vi "prueba2.vi"() -> ()   [LabVIEW 2016]
uses:
  C:/Users/Polaritones IICO/Desktop/Camara y mapeo/rot/Thorlabs.MotionControl.Controls.dll
  rot/Thorlabs.MotionControl.Controls.dll
  <vilib>/userdefined/High Color/IMAQdx.ctl
  <vilib>/UPVI/lvhdf5/file.llb/LVH5F Operation.ctl
  C:/Users/Polaritones IICO/Desktop/Camara y mapeo/rot/Thorlabs.MotionControl.IntegratedStepperMotorsCLI.dll
  rot/Thorlabs.MotionControl.IntegratedStepperMotorsCLI.dll
  <vilib>/Utility/miscctls.llb/LVRectTypeDef.ctl
  <vilib>/UPVI/lvhdf5/group.llb/H5G_obj_t.ctl
  <vilib>/UPVI/lvhdf5/dataset.llb/LVH5D Operation.ctl
  <vilib>/Analysis/baseanly.llb/Mean (DBL).vi
  <vilib>/UPVI/lvhdf5/group.llb/OpenCreateGroup (String).vi
  <vilib>/UPVI/lvhdf5/utility.llb/Select HDF5 Dialog.vi
  <vilib>/UPVI/lvhdf5/utility.llb/Select HDF5 Dialog (Object Only).vi
  <vilib>/UPVI/lvhdf5/dataset.llb/Simple H5Dwrite (Variant).vi
  <vilib>/UPVI/lvhdf5/library.llb/HDF5 Ref.ctl
  <vilib>/UPVI/lvhdf5/dataset.llb/Simple H5Dwrite.xnode
  <vilib>/vision/driver/NI_Vision_Acquisition_Software.lvlib
  <instrlib>/Keithley 2200 Series/Keithley 2200 Series.lvlib
  <vilib>/Analysis/NI_AALBase.lvlib
  <vilib>/UPVI/lvhdf5/identifier.llb/Not an HDF5 Refnum Constant.vi
  <vilib>/Utility/error.llb/Error Cluster From Error Code.vi
  <vilib>/UPVI/lvhdf5/dataset.llb/OpenCreateReplace Dataset by Element Type.vi
  <vilib>/UPVI/lvhdf5/dataspace.llb/H5Sselect_hyperslab.vi
  <vilib>/UPVI/lvhdf5/dataset.llb/H5Dwrite (Variant).vi
  <vilib>/UPVI/lvhdf5/dataset.llb/H5Dget_space.vi
  <vilib>/UPVI/lvhdf5/attribute.llb/private/LVH5AwriteWDTAttrs.vi
  <vilib>/UPVI/lvhdf5/dataspace.llb/H5Sclose.vi
  <vilib>/UPVI/lvhdf5/dataset.llb/H5Dclose.vi
  <vilib>/UPVI/lvhdf5/utility.llb/Select HDF5 Dialog (File and Object).vi
panel:
  out "valor potenciometro":dbl format="%^#_9e"
  out "Readout string":string
  out "New":bool
  out "Error log":string
  in  "path":path
  out "Ángulo del polarizador":i32
  in  "CageRotatorControl":refnum<k24>(container)
  in  "SerialNumber":string="55000538"
  in  "Ring":u16(ring)
  out "I-V":cluster{dbl[], dbl[]}(graph)
  out "corriente":dbl
  in  "stop medición":bool
  in  "stop":bool
  in  "Iniciar medición":bool
  out "LockIn":dbl
  out "Valor voltaje":dbl
  in  "Config. fotodiodo":cluster{"tiempo. lect.":dbl, "num. med":dbl}
  in  "Powermeter":T1={"Readout Config"="POW", "tiempo. lect."=0.0, "average rate"=0.0}
  in  "config. Polarizador":T2
  in  "Config. voltaje y corriente":T3 {"Measurement Function (0:Voltage)" items=["Voltage", "Current", "Power"]; "Unit(V)" items=["V", "mV", "kV", "A", "mA"]; "Function(0:Voltage)" items=["Voltage", "Current"]}
  in  "yFin":dbl
  in  "Paso":dbl=0.01
  in  "xFin":dbl
  in  "Movimiento de spot en x":ext(slide) scale=-10.0..10.0
  in  "Movimiento de spot en y":dbl(slide) min=-10.0 max=10.0 scale=-10.0..10.0
  out "xsal":dbl
  out "ysal":dbl
  in  "tipo":enum16{"barrido", "manual"}(ring)
  out "Fototubo":cluster{dbl[], dbl[]}(graph)
  out "Power meter":cluster{dbl[], dbl[]}(graph)
  out "Imágen":T4(plugin-control)
  # "Control espejos"
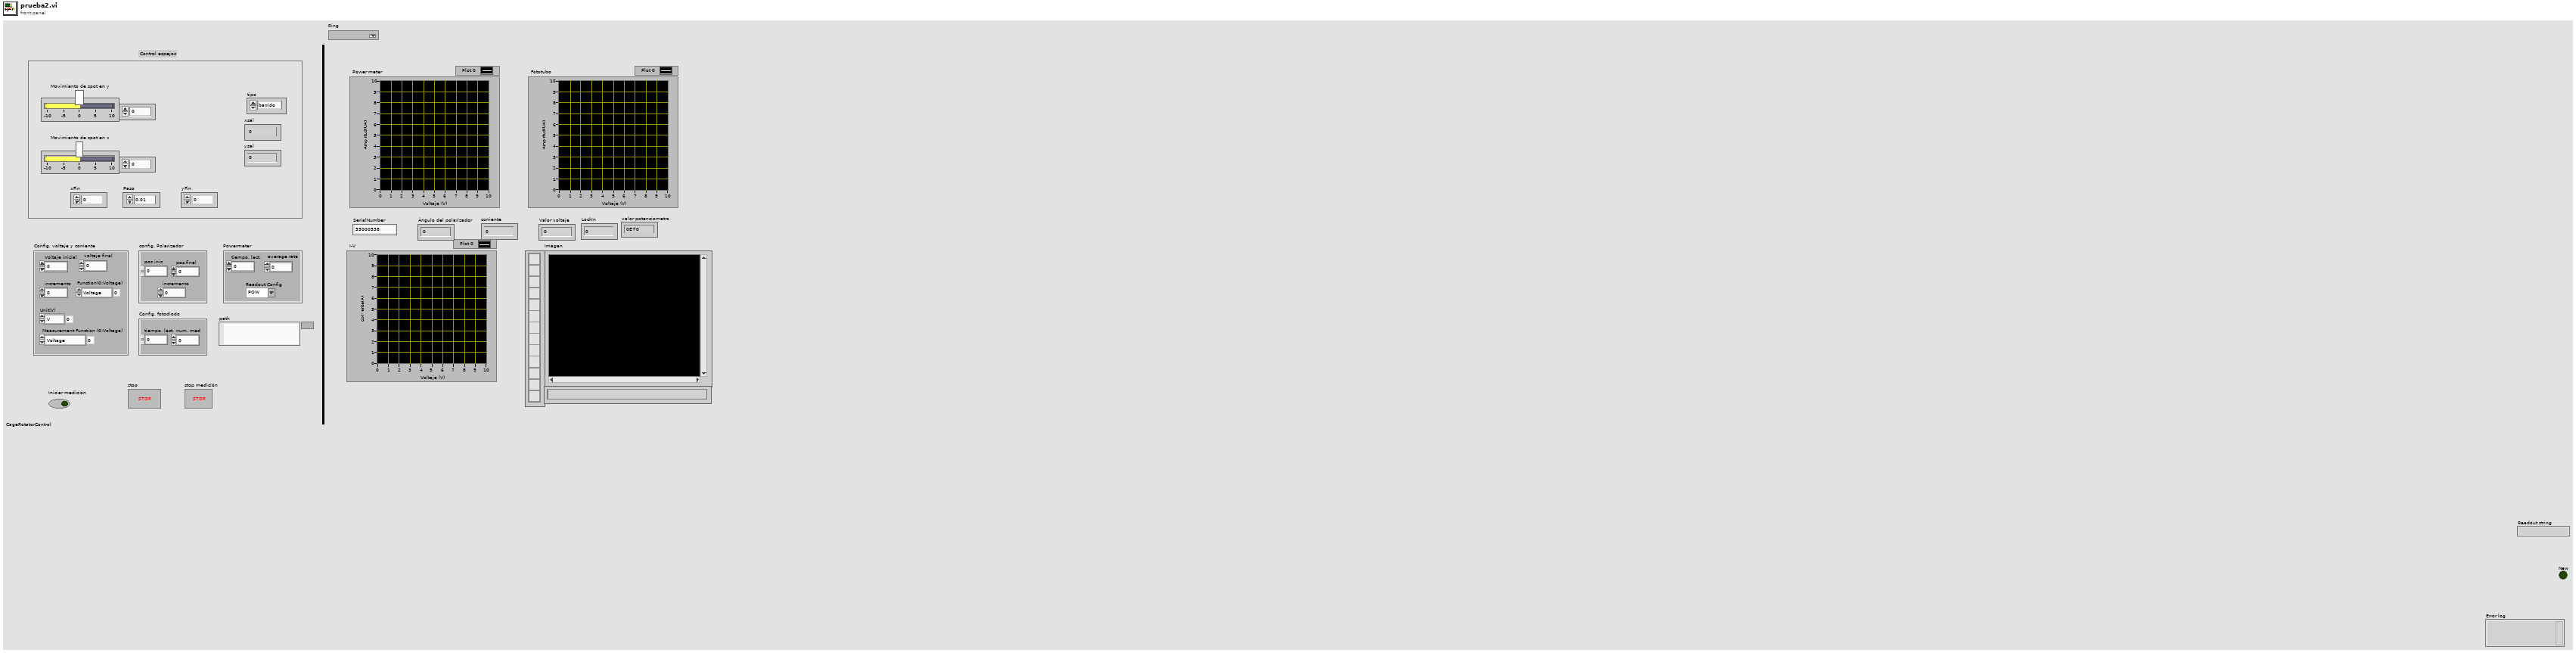
[diagram p1: front panel]
types:
  T1 = cluster{"Readout Config":string, "tiempo. lect.":dbl, "average rate":dbl}
  T2 = cluster{"pos inic":dbl, "pos.final":dbl, "incremento":dbl}
  T3 = cluster{"Voltaje inicial":dbl, "incremento":dbl, " voltaje final":dbl, "Function(0:Voltage)":u16, "Unit(V)":u16, "Measurement Function (0:Voltage)":u16}
  T4 = typedef "IMAQ Image.ctl" = refnum<image>
  T5 = typedef "IMAQdx.ctl" = refnum<k21>
  T6 = typedef "LVH5F Operation.ctl" = enum16{"open", "open or create", "create or replace", "create or replace (with confirmation)", "create", "open (read only)"}
  T7 = typedef "LVRectTypeDef.ctl" = cluster{"Left":i16, "Top":i16, "Right":i16, "Bottom":i16}
  T8 = cluster{"Behavior":enum32{"Invalid", "Default", "Floating", "Floating/Auto-Hide", "Modal"}, "Position":T7, "Center":bool, "Title":string}
  T9 = typedef "LVH5D Operation.ctl" = enum16{"open", "replace", "create", "open or create", "create or replace", "create or replace with confirmation"}
  T10 = typedef "H5G_obj_t.ctl" = i32
  T11 = cluster{"Object Types (any)":T10[], "Object Pattern":string}
  T12 = typedef "Image Type" = u32
  T13 = typedef "HDF5 Ref.ctl" = refnum<k1>
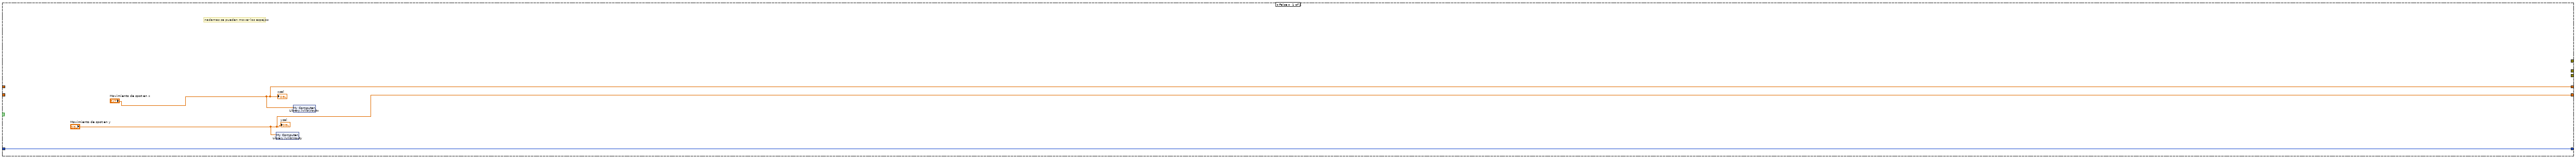
[diagram p2: hidden frame]
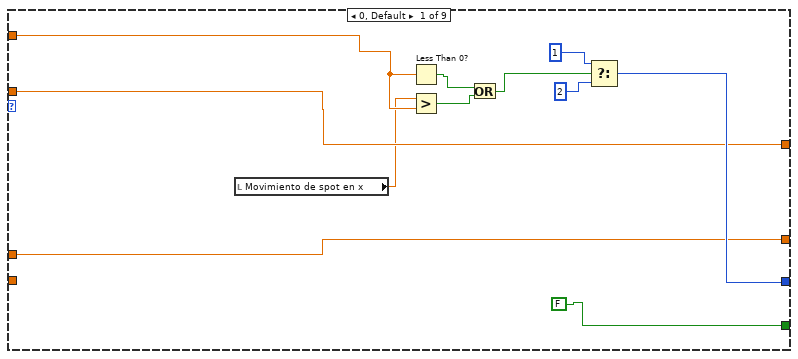
[diagram p3: hidden frame]
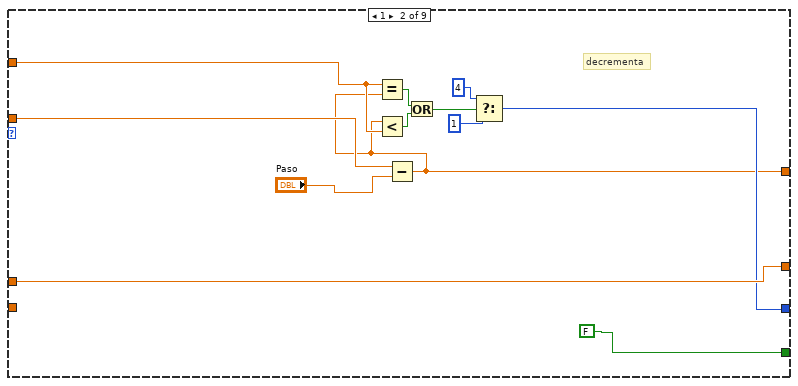
[diagram p4: hidden frame]
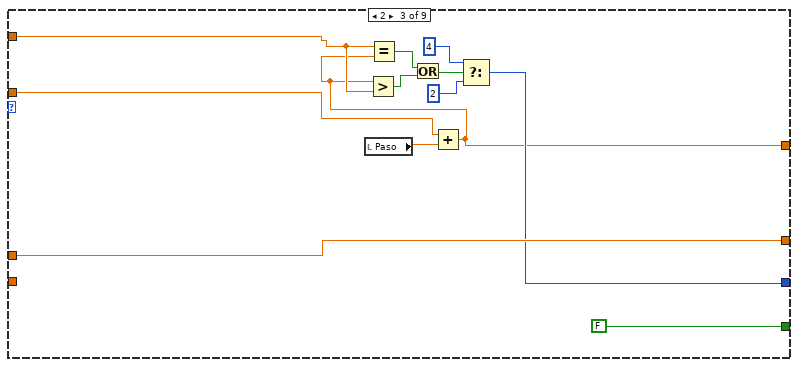
[diagram p5: hidden frame]
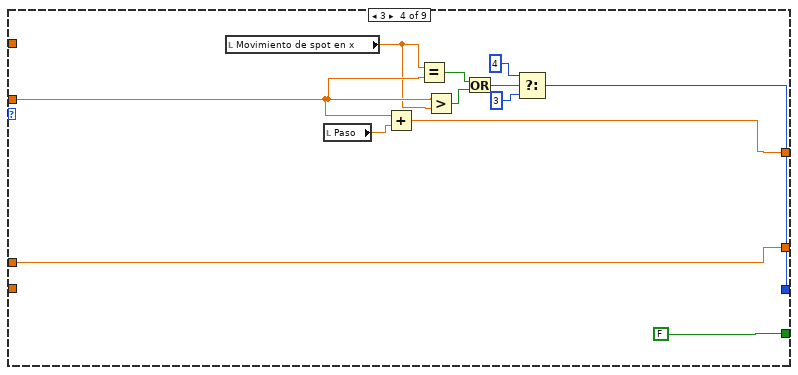
[diagram p6: hidden frame]
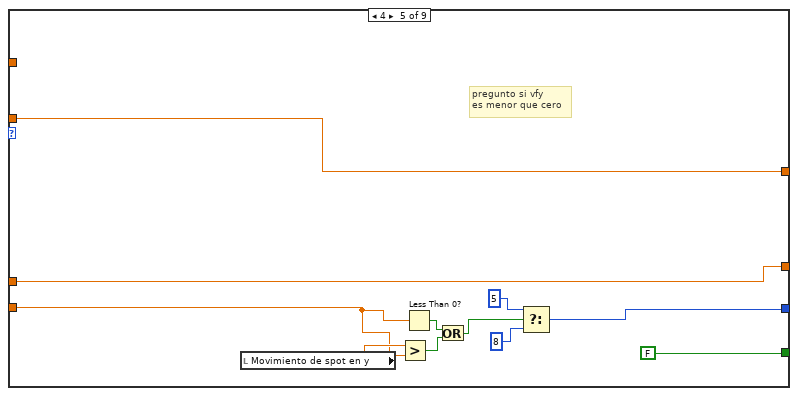
[diagram p7: hidden frame]
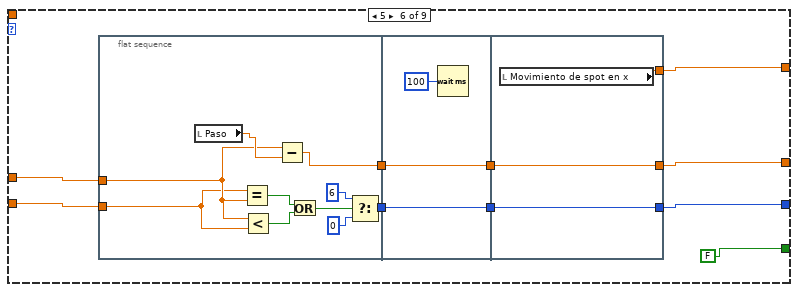
[diagram p8: hidden frame]
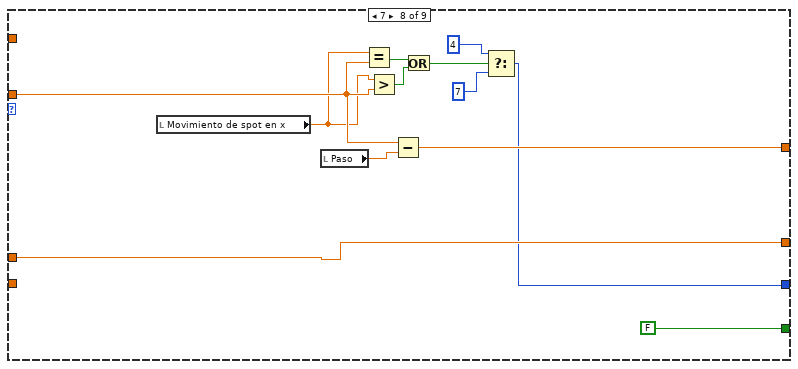
[diagram p9: hidden frame]
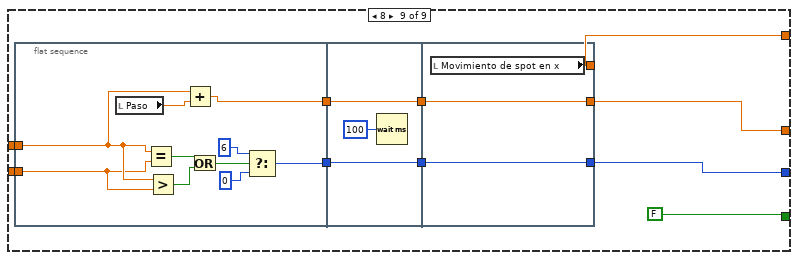
[diagram p10: hidden frame]
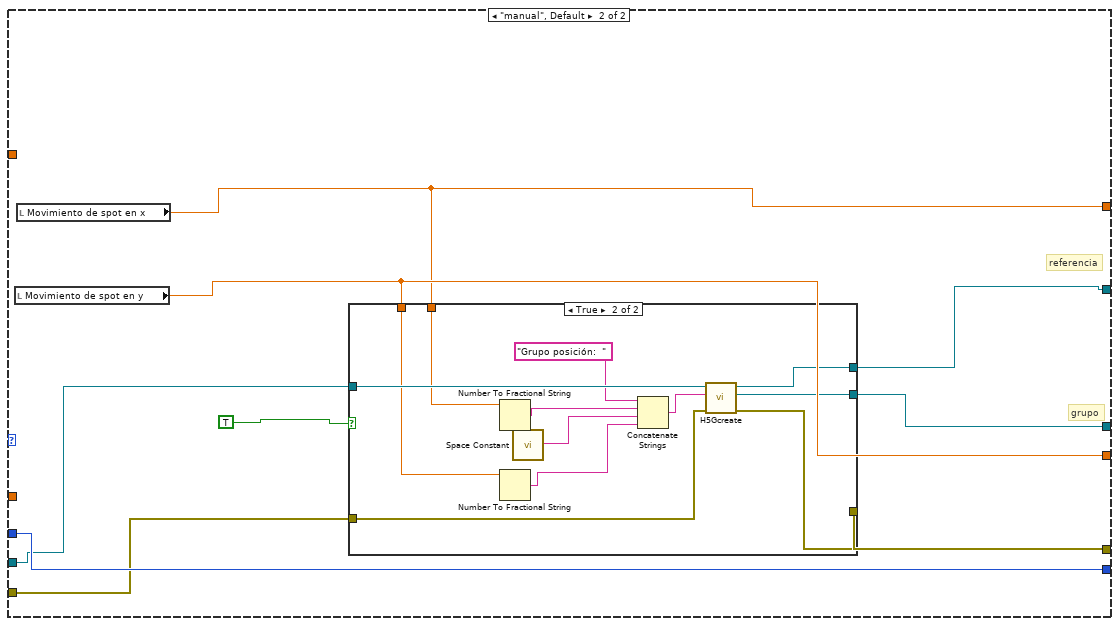
[diagram p11: hidden frame]
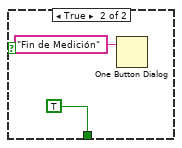
[diagram p14: hidden frame]
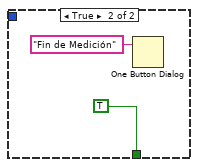
[diagram p15: hidden frame]
diagram:
  n1 = flat-sequence {
    tunnel: [w15] -> w12
    tunnel: [w14] -> w11
    tunnel: [w13] -> w10
    tunnel: w12 -> [w32]
    tunnel: w11 -> [w31]
    tunnel: w10 -> [w30]
    tunnel: [w28] -> w4
    tunnel: [w27] -> w3
    tunnel: [w26] -> w2
    tunnel: [w25] -> _
    tunnel: [w24] -> w7
    tunnel: [w23] -> w6
    tunnel: [w22] -> w8
    frame #0 {
      w17 = T12 4 items=["Grayscale (U8)", "Grayscale (I16)", "Grayscale (SGL)", "Complex (CSG)", "RGB (U32)", "HSL (U32)", "RGB (U64)", "Grayscale (U16)"] ("Image Type")
      w21 = 5.0
      # "inicializar espejos"
      n2 = call <vilib>:"IMAQdx Open Camera.vi"("Session In"=T5 "cam0") -> ("error out"=w19:errorcluster, "Session Out"=w20:T5)  [unwired: 9 in]
      n3 = call "IMAQ Create"("Image Name"="imagen", "Image Type"=w17) -> ("New Image"=w15:T4)  [unwired: 3 in, 1 out]
      n4 = call <vilib>:"IMAQdx Configure Grab.vi"("error in"=w19, "Session In"=w20) -> ("error out"=w13:errorcluster, "Session Out"=w14:T5)  [unwired: 8 in]
      n5 = shared-variable "My Computer\\Library.lvlib\\Voutx"(w21) -> ()  [unwired: 1 in, 1 out]
      n6 = shared-variable "My Computer\\Library.lvlib\\Vouty"(w21) -> ()  [unwired: 1 in, 1 out]
    }
    frame #1 {
      # "programa en ejecución"
      n7 = while {
        shift-right: [w48] -> _
        shift-left: _ -> [w46]
        shift-right: [w47] -> _
        shift-left: _ -> [w45]
        shift-right: [w38] -> _
        shift-left: 0 -> [w37]
        tunnel: w32 -> [w42]
        tunnel: w31 -> [w44]
        tunnel: w30 -> [w43]
        tunnel: [w41] -> w22
        tunnel: [w40] -> w23
        tunnel: [w39] -> w24
        tunnel: [w36] -> w28
        tunnel: [w35] -> w27
        tunnel: [w34] -> w26
        tunnel: [w33] -> w25
        stop <- "stop" stop-if-true
        n8 = case shown="True" "Iniciar medición" {
          tunnel: ["Movimiento de spot en x" w70] -> w48
          tunnel: ["Movimiento de spot en y" w69] -> w47
          tunnel: w46 -> [_ w73]
          tunnel: w45 -> [_ w71]
          tunnel: [w51 w65] -> w38
          tunnel: w37 -> [w51 w63]
          tunnel: [_ w60] -> w36
          tunnel: [_ w59] -> w35
          tunnel: [_ w57] -> w34
          tunnel: [_ w55] -> w33
          frame False {
            # "nadamas se pueden mover los espejos"
            n9 = shared-variable "My Computer\\Library.lvlib\\Vouty"("Movimiento de spot en y") -> ()  [unwired: 1 in, 1 out]
            n10 = shared-variable "My Computer\\Library.lvlib\\Voutx"("Movimiento de spot en x") -> ()  [unwired: 1 in, 1 out]
            "xsal" <- "Movimiento de spot en x"
            "ysal" <- "Movimiento de spot en y"
          }
          frame True {
            n11 = flat-sequence {
              tunnel: [w81] -> w76
              tunnel: [w80] -> w75
              tunnel: [w79] -> w74
              tunnel: w73 -> [w79]
              tunnel: [w78] -> w72
              tunnel: w71 -> [w78]
              tunnel: [w77] -> w64
              tunnel: w63 -> [w77]
              tunnel: w76 -> [w90]
              tunnel: w75 -> [w89]
              tunnel: w74 -> [w96]
              tunnel: w72 -> [w95]
              tunnel: [w94] -> w68
              tunnel: [w93] -> w67
              tunnel: [w92] -> w66
              tunnel: w64 -> [w91]
              tunnel: [w88] -> w62
              tunnel: [w87] -> w61
              tunnel: [w86] -> w58
              tunnel: [w85] -> w56
              tunnel: [w84] -> w54
              tunnel: [w920] -> w69
              tunnel: [w921] -> w70
              tunnel: w68 -> [w921]
              tunnel: w67 -> [w920]
              tunnel: w66 -> [w919]
              tunnel: [w919] -> w65
              tunnel: w62 -> [w918]
              tunnel: w61 -> [w917]
              tunnel: [w916] -> w60
              tunnel: [w915] -> w59
              tunnel: w58 -> [w915]
              tunnel: [w914] -> w57
              tunnel: w56 -> [w914]
              tunnel: [w913] -> w55
              tunnel: w54 -> [w913]
              frame #0 {
                # "abrir archivo"
                n12 = call <vilib>:"OpenCreateReplace HDF5 File.vi"("function (open or create)"=LVH5F_Operation."open or create", "path"="path") -> ("error out"=w80:errorcluster, "HDF5 Ref out"=w81:T13)  [unwired: 6 in]
              }
              frame #1 {
                n13 = while {
                  shift-right: [w114] -> w94
                  shift-left: w96 -> [w122]
                  shift-right: [w115] -> w93
                  shift-left: w95 -> [w121]
                  shift-right: [w123] -> w92
                  shift-left: w91 -> [w124]
                  tunnel: w90 -> [w126]
                  tunnel: w89 -> [w125]
                  tunnel: [w101] -> w88
                  tunnel: [w100] -> w87
                  tunnel: [w99] -> w86
                  tunnel: [w98] -> w85
                  tunnel: [w97] -> w84
                  stop <- w107 stop-if-true
                  n14 = flat-sequence {
                    tunnel: w126 -> [w138]
                    tunnel: w125 -> [w137]
                    tunnel: w124 -> [w136]
                    tunnel: w122 -> [w134]
                    tunnel: w121 -> [w133]
                    tunnel: [w135] -> w120
                    tunnel: [w132] -> w119
                    tunnel: [w131] -> w118
                    tunnel: [w130] -> w117
                    tunnel: [w129] -> w116
                    tunnel: [w127] -> w113
                    tunnel: w120 -> [w325]
                    tunnel: w119 -> [w329]
                    tunnel: w118 -> [w323]
                    tunnel: w117 -> [w328]
                    tunnel: w116 -> [w327]
                    tunnel: w113 -> [w322]
                    tunnel: [w325] -> w112
                    tunnel: [w329] -> w111
                    tunnel: [w328] -> w110
                    tunnel: [w327] -> w109
                    tunnel: [w321] -> w105
                    tunnel: [w320] -> w104
                    tunnel: [w319] -> w103
                    tunnel: [w318] -> w102
                    tunnel: [w901] -> w115
                    tunnel: [w902] -> w114
                    tunnel: [w903] -> w100
                    tunnel: [w896] -> w123
                    tunnel: w112 -> [w896]
                    tunnel: w111 -> [w903]
                    tunnel: w110 -> [w902]
                    tunnel: w109 -> [w901]
                    tunnel: [w897] -> w106
                    tunnel: [w895] -> w98
                    tunnel: w105 -> [w895]
                    tunnel: [w894] -> w99
                    tunnel: w104 -> [w894]
                    tunnel: [w893] -> w97
                    tunnel: w103 -> [w893]
                    tunnel: [w892] -> w101
                    tunnel: w102 -> [w892]
                    frame #0 {
                      # "barrido"
                      n15 = case shown="\"barrido\"" "tipo" {
                        tunnel: [w142 w296] -> w130
                        tunnel: [w141 w297] -> w129
                        tunnel: w136 -> [w156 w303]
                        tunnel: w134 -> [w155 _]
                        tunnel: w133 -> [w154 _]
                        tunnel: [w153 w303] -> w135
                        tunnel: w138 -> [w147 w302]
                        tunnel: [w144 w301] -> w131
                        tunnel: [w145 w300] -> w132
                        tunnel: w137 -> [w146 w299]
                        tunnel: [w143 w298] -> w127
                        frame "barrido" {
                          n16 = flat-sequence {
                            tunnel: "xFin" -> [w165]
                            tunnel: w156 -> [w164]
                            tunnel: [w163] -> w142
                            tunnel: [w162] -> w141
                            tunnel: "yFin" -> [w161]
                            tunnel: w155 -> [w160]
                            tunnel: w154 -> [w159]
                            tunnel: [w158] -> w153
                            tunnel: [w157] -> _
                            frame #0 {
                              n17 = case shown="6" w164 {
                                tunnel: w160 -> [w172 w184 w198 w210 w223 _ w256 w259 _]
                                tunnel: w165 -> [w171 w183 w197 _ _ _ _ _ _]
                                tunnel: w159 -> [w173 w188 w200 w202 w222 w231 w255 w268 w276]
                                tunnel: w161 -> [_ _ _ _ w217 w230 _ _ w275]
                                tunnel: [w175 w185 w193 w204 w220 w233 w253 w265 w277] -> w158
                                tunnel: [w173 w188 w200 w202 w222 w232 w255 w268 w278] -> w162
                                tunnel: [w172 w179 w190 w211 w223 w228 w256 w266 w273] -> w163
                                tunnel: [FALSE FALSE FALSE FALSE ("true") FALSE ("true") FALSE FALSE FALSE ("true") FALSE] -> w157
                                frame 0, Default {
                                n18 = local read "Movimiento de spot en x"() -> (w167:ext)
                                n19 = Less Than 0?(x=w171) -> (x < 0?=w169:bool)
                                n20 = Greater?(x=w167, y=w171) -> (0:w170:bool)
                                n21 = Or(x=w169, y=w170) -> (x .or. y?=w168:bool)
                                n22 = Select(t=1, s=w168, f=2) -> (s? t:f=w175:i32)
                                }
                                frame 1 {
                                # "decrementa"
                                n23 = Subtract(x=w184, y="Paso") -> (x-y=w179:ext)
                                n24 = Equal?(x=w183, y=w179) -> (x = y?=w181:bool)
                                n25 = Less?(x=w179, y=w183) -> (x < y?=w182:bool)
                                n26 = Or(x=w181, y=w182) -> (x .or. y?=w180:bool)
                                n27 = Select(t=4, s=w180, f=1) -> (s? t:f=w185:i32)
                                }
                                frame 2 {
                                n28 = local read "Paso"() -> (w199:dbl)
                                n29 = Add(x=w198, y=w199) -> (x+y=w190:ext)
                                n30 = Greater?(x=w190, y=w197) -> (0:w196:bool)
                                n31 = Equal?(x=w197, y=w190) -> (x = y?=w195:bool)
                                n32 = Or(x=w195, y=w196) -> (x .or. y?=w194:bool)
                                n33 = Select(t=4, s=w194, f=2) -> (s? t:f=w193:i32)
                                }
                                frame 3 {
                                n34 = local read "Movimiento de spot en x"() -> (w209:ext)
                                n35 = local read "Paso"() -> (w212:dbl)
                                n36 = Add(x=w210, y=w212) -> (x+y=w211:ext)
                                n37 = Equal?(x=w209, y=w210) -> (x = y?=w207:bool)
                                n38 = Greater?(x=w210, y=w209) -> (0:w208:bool)
                                n39 = Or(x=w207, y=w208) -> (x .or. y?=w206:bool)
                                n40 = Select(t=4, s=w206, f=3) -> (s? t:f=w204:i32)
                                }
                                frame 4 {
                                # "pregunto si vfy\nes menor que cero"
                                n41 = local read "Movimiento de spot en y"() -> (w218:dbl)
                                n42 = Greater?(x=w218, y=w217) -> (0:w215:bool)
                                n43 = Less Than 0?(x=w217) -> (x < 0?=w216:bool)
                                n44 = Or(x=w216, y=w215) -> (x .or. y?=w214:bool)
                                n45 = Select(t=5, s=w214, f=8) -> (s? t:f=w220:i32)
                                }
                                frame 5 {
                                n46 = flat-sequence {
                                tunnel: w231 -> [w236]
                                tunnel: w230 -> [w235]
                                tunnel: [w241] -> w227
                                tunnel: [w239] -> w225
                                tunnel: w227 -> [w246]
                                tunnel: [w246] -> w226
                                tunnel: w225 -> [w245]
                                tunnel: [w245] -> w224
                                tunnel: [w248] -> w232
                                tunnel: [w249] -> w233
                                tunnel: w226 -> [w249]
                                tunnel: w224 -> [w248]
                                tunnel: [w247] -> w228
                                frame #0 {
                                n47 = local read "Paso"() -> (w240:dbl)
                                n48 = Equal?(x=w235, y=w236) -> (x = y?=w237:bool)
                                n49 = Less?(x=w236, y=w235) -> (x < y?=w234:bool)
                                n50 = Subtract(x=w236, y=w240) -> (x-y=w239:dbl)
                                n51 = Or(x=w237, y=w234) -> (x .or. y?=w238:bool)
                                n52 = Select(t=6, s=w238, f=0) -> (s? t:f=w241:i32)
                                }
                                frame #1 {
                                n53 = Wait (ms)(milliseconds to wait=u32 100) -> ()  [unwired: 1 out]
                                }
                                frame #2 {
                                n54 = local read "Movimiento de spot en x"() -> (w247:ext)
                                }
                                }
                                }
                                frame 6 {
                                # "stop"
                                n55 = Select(t=0, s=TRUE, f=6) -> (s? t:f=w253:i32)
                                }
                                frame 7 {
                                n56 = local read "Movimiento de spot en x"() -> (w257:ext)
                                n57 = local read "Paso"() -> (w267:dbl)
                                n58 = Equal?(x=w257, y=w259) -> (x = y?=w264:bool)
                                n59 = Greater?(x=w257, y=w259) -> (0:w260:bool)
                                n60 = Subtract(x=w259, y=w267) -> (x-y=w266:ext)
                                n61 = Or(x=w264, y=w260) -> (x .or. y?=w263:bool)
                                n62 = Select(t=4, s=w263, f=7) -> (s? t:f=w265:i32)
                                }
                                frame 8 {
                                n63 = flat-sequence {
                                tunnel: w276 -> [w281]
                                tunnel: w275 -> [w280]
                                tunnel: [w287] -> w272
                                tunnel: [w283] -> w270
                                tunnel: w272 -> [w291]
                                tunnel: [w291] -> w271
                                tunnel: w270 -> [w290]
                                tunnel: [w290] -> w269
                                tunnel: [w293] -> w277
                                tunnel: [w294] -> w278
                                tunnel: w271 -> [w294]
                                tunnel: w269 -> [w293]
                                tunnel: [w292] -> w273
                                frame #0 {
                                n64 = local read "Paso"() -> (w288:dbl)
                                n65 = Equal?(x=w281, y=w280) -> (x = y?=w286:bool)
                                n66 = Greater?(x=w281, y=w280) -> (0:w282:bool)
                                n67 = Add(x=w281, y=w288) -> (x+y=w287:dbl)
                                n68 = Or(x=w286, y=w282) -> (x .or. y?=w285:bool)
                                n69 = Select(t=6, s=w285, f=0) -> (s? t:f=w283:i32)
                                }
                                frame #1 {
                                n70 = Wait (ms)(milliseconds to wait=u32 100) -> ()  [unwired: 1 out]
                                }
                                frame #2 {
                                n71 = local read "Movimiento de spot en x"() -> (w292:ext)
                                }
                                }
                                }
                              }
                            }
                          }
                          n72 = Number To Fractional String(number=w142) -> (F-format string=w150:string)  [unwired: 3 in]
                          n73 = Number To Fractional String(number=w141) -> (F-format string=w148:string)  [unwired: 3 in]
                          n74 = call <vilib>:"Space Constant.vi"() -> ("String"=w149:string)
                          n75 = Concatenate Strings("Grupo posición:  " ("string"), w150, w149, w148) -> (w152:string)
                          n76 = call-poly <vilib>:"OpenCreateGroup.vi"("error in (no error)"=w146, "Group"=w152, "HDF5 Ref"=w147) -> ("error out"=w143:errorcluster, "HDF5 Group Ref"=w144:T13, "HDF5 Ref out"=w145:T13)  [unwired: 6 in]
                        }
                        frame "manual", Default {
                          # "referencia"
                          # "grupo"
                          n77 = local read "Movimiento de spot en y"() -> (w297:dbl)
                          n78 = local read "Movimiento de spot en x"() -> (w296:ext)
                          n79 = case shown="True" TRUE {
                            tunnel: w302 -> [w305 w317]
                            tunnel: [_ w316] -> w301
                            tunnel: [w305 w315] -> w300
                            tunnel: w296 -> [_ w312]
                            tunnel: w297 -> [_ w309]
                            tunnel: w299 -> [w304 w307]
                            tunnel: [w304 w306] -> w298
                            frame False {
                            }
                            frame True {
                              n80 = Number To Fractional String(number=w312) -> (F-format string=w311:string)  [unwired: 3 in]
                              n81 = Number To Fractional String(number=w309) -> (F-format string=w308:string)  [unwired: 3 in]
                              n82 = call <vilib>:"Space Constant.vi"() -> ("String"=w310:string)
                              n83 = Concatenate Strings("Grupo posición:  " ("string"), w311, w310, w308) -> (w314:string)
                              n84 = call <vilib>:"H5Gcreate.vi"("error in (no error)"=w307, "Name"=w314, "HDF5 Ref"=w317) -> ("error out"=w306:errorcluster, "HDF5 Group Ref"=w316:T13, "HDF5 Ref out"=w315:T13)  [unwired: 4 in]
                            }
                          }
                        }
                      }
                      n85 = local write "xsal"(w130) -> ()
                      n86 = shared-variable "My Computer\\Library.lvlib\\Voutx"(w130) -> ()  [unwired: 1 in, 1 out]
                      n87 = local write "ysal"(w129) -> ()
                      n88 = shared-variable "My Computer\\Library.lvlib\\Vouty"(w129) -> ()  [unwired: 1 in, 1 out]
                    }
                    frame #1 {
                      n89 = Not Equal?(x=w325, y=4) -> (x != y?=w326:bool)
                      n90 = case shown="True" w326 {
                        tunnel: w323 -> [_ w347]
                        tunnel: w322 -> [_ w342]
                        tunnel: [_ w333] -> w321
                        tunnel: [_ w332] -> w320
                        tunnel: [_ w331] -> w319
                        tunnel: [_ w330] -> w318
                        frame False {
                        }
                        frame True {
                          n91 = flat-sequence {
                            tunnel: [w377] -> w364
                            tunnel: [w376] -> w363
                            tunnel: [w370] -> w362
                            tunnel: [w368] -> w361
                            tunnel: [w367] -> w356
                            tunnel: w347 -> [w366]
                            tunnel: [w366] -> w345
                            tunnel: [w365] -> w343
                            tunnel: w342 -> [w365]
                            tunnel: w364 -> [w389]
                            tunnel: w363 -> [w388]
                            tunnel: w362 -> [w387]
                            tunnel: w361 -> [w386]
                            tunnel: [w389] -> w360
                            tunnel: [w388] -> w359
                            tunnel: [w384] -> w358
                            tunnel: [w383] -> w357
                            tunnel: w356 -> [w383]
                            tunnel: [w382] -> w355
                            tunnel: [w381] -> w346
                            tunnel: w345 -> [w381]
                            tunnel: w343 -> [w380]
                            tunnel: [w380] -> w340
                            tunnel: w360 -> [w411]
                            tunnel: w359 -> [w410]
                            tunnel: w358 -> [w396]
                            tunnel: w357 -> [w401]
                            tunnel: w355 -> [w395]
                            tunnel: [w411] -> w354
                            tunnel: [w410] -> w353
                            tunnel: [w405] -> w352
                            tunnel: [w401] -> w351
                            tunnel: [w400] -> w350
                            tunnel: [w393] -> w349
                            tunnel: [w392] -> w348
                            tunnel: w346 -> [w391]
                            tunnel: [w391] -> w344
                            tunnel: [w390] -> w341
                            tunnel: w340 -> [w390]
                            tunnel: w354 -> [w420]
                            tunnel: w353 -> [w419]
                            tunnel: w352 -> [w417]
                            tunnel: w351 -> [w425]
                            tunnel: w350 -> [w424]
                            tunnel: w349 -> [w423]
                            tunnel: w348 -> [w422]
                            tunnel: w344 -> [w421]
                            tunnel: w341 -> [w418]
                            tunnel: [w425] -> w339
                            tunnel: [w416] -> w338
                            tunnel: [w415] -> w337
                            tunnel: [w414] -> w336
                            tunnel: [w413] -> w335
                            tunnel: [w412] -> w334
                            tunnel: w339 -> [w890]
                            tunnel: w338 -> [w891]
                            tunnel: [w889] -> w331
                            tunnel: [w888] -> w333
                            tunnel: w337 -> [w888]
                            tunnel: [w887] -> w332
                            tunnel: w336 -> [w887]
                            tunnel: w335 -> [w886]
                            tunnel: w334 -> [w885]
                            tunnel: [w884] -> w330
                            frame #0 {
                              # "polarizador"
                              # "potenciometro"
                              # "Configurar aparatos"
                              n92 = property class="CageRotatorControl"(reference="CageRotatorControl", "SerialNumber"="SerialNumber") -> (reference out=w375:refnum<k24>, error out=w374:errorcluster)  [unwired: 1 in]
                              n93 = call "PM100D_Initialize.vi"() -> ("error out"=w379:errorcluster, "VISA out"=w378:refnum<visa-resource-name>)  [unwired: 2 in, 2 out]
                              n94 = invoke class="CageRotatorControl" method="CreateDevice"(reference=w375, error in=w374) -> (reference out=w373:refnum<k24>, error out=w372:errorcluster)  [unwired: 1 in, 1 out]
                              n95 = call "PM100D_SensorFlag.vi"("error in (no error)"=w379, "VISA in"=w378) -> ("error out"=w376:errorcluster, "VISA out"=w377:refnum<visa-resource-name>)  [unwired: 2 in, 6 out]
                              n96 = property class="CageRotatorControl"(reference=w373, error in=w372) -> (reference out=w367:refnum<k24>, error out=w368:errorcluster, "Device"=w370:refnum<k24>)
                            }
                            frame #1 {
                              # "timeout polarizador"
                              n97 = invoke class="IntegratedStepperMotor" method="Home"(reference=w387, error in=w386, "waitTimeout"=10000) -> (reference out=w384:refnum<k24>, error out=w382:errorcluster)  [unwired: 1 in, 2 out]
                            }
                            frame #2 {
                              # "inicializa polarizador\ny parametros de medición."
                              n98 = local read "config. Polarizador"() -> (w404:T2)
                              n99 = Unbundle By Name(w404) -> ("pos inic"=w394:dbl, "pos.final"=w403:dbl, "incremento"=w402:dbl)
                              n100 = invoke class="IntegratedStepperMotor" method="SetMoveAbsolutePosition"(reference=w396, error in=w395, "position"=w394) -> (reference out=w399:refnum<k24>, error out=w397:errorcluster)  [unwired: 1 in, 2 out]
                              n101 = local read "Config. voltaje y corriente"() -> (w409:T3)
                              n102 = Unbundle By Name(w409) -> ("Voltaje inicial"=w408:dbl, "incremento"=w407:dbl, "voltaje final"=w406:dbl)
                              n103 = call "intervalo.vi"("incremento"=w402, "fin"=w403, "inicio"=w394) -> ("Array"=w400:dbl[])  [unwired: 8 in]
                              n104 = call "intervalo.vi"("incremento"=w407, "fin"=w406, "inicio"=w408) -> ("Array"=w405:dbl[])  [unwired: 8 in]
                              n105 = invoke class="IntegratedStepperMotor" method="MoveAbsolute"(reference=w399, error in=w397, "waitTimeout"=0) -> (reference out=w393:refnum<k24>, error out=w392:errorcluster)  [unwired: 1 in, 2 out]
                            }
                            frame #3 {
                              # "parte de l barrido del polarizador"
                              n106 = for {
                                tunnel: w424 -> [w454] mode=indexing
                                tunnel: w423 -> [w456]
                                tunnel: w422 -> [w455]
                                tunnel: w421 -> [w453]
                                tunnel: w420 -> [w443]
                                tunnel: w419 -> [w441]
                                tunnel: w418 -> [w452]
                                tunnel: w417 -> [w446]
                                tunnel: [w430] -> w416
                                tunnel: [w429] -> w415
                                tunnel: [w428] -> w414
                                tunnel: [w427] -> w413
                                tunnel: [w426] -> w412
                                stop <- "stop medición" stop-if-true
                                n107 = flat-sequence {
                                tunnel: w456 -> [w480]
                                tunnel: w455 -> [w479]
                                tunnel: w454 -> [w466]
                                tunnel: w453 -> [w465]
                                tunnel: w452 -> [w464]
                                tunnel: [w473] -> w451
                                tunnel: [w472] -> w450
                                tunnel: [w463] -> w449
                                tunnel: [w462] -> w448
                                tunnel: [w461] -> w447
                                tunnel: w446 -> [w461]
                                tunnel: [w460] -> w445
                                tunnel: [w459] -> w444
                                tunnel: w443 -> [w459]
                                tunnel: [w458] -> w442
                                tunnel: w441 -> [w458]
                                tunnel: w451 -> [_]
                                tunnel: w450 -> [w487]
                                tunnel: w449 -> [w485]
                                tunnel: w448 -> [w486]
                                tunnel: w447 -> [w494]
                                tunnel: w445 -> [w490]
                                tunnel: w444 -> [w492]
                                tunnel: w442 -> [w491]
                                tunnel: [w490] -> w440
                                tunnel: [w489] -> w439
                                tunnel: [w488] -> w438
                                tunnel: [w487] -> w437
                                tunnel: [w486] -> w436
                                tunnel: [w485] -> w435
                                tunnel: [w484] -> w434
                                tunnel: [w483] -> w433
                                tunnel: [w482] -> w432
                                tunnel: [w481] -> w431
                                tunnel: w440 -> [w681]
                                tunnel: [w681] -> w426
                                tunnel: [w680] -> w428
                                tunnel: w439 -> [w680]
                                tunnel: [w679] -> w429
                                tunnel: w438 -> [w679]
                                tunnel: [w678] -> w430
                                tunnel: w437 -> [w678]
                                tunnel: w436 -> [w669]
                                tunnel: w435 -> [w670]
                                tunnel: w434 -> [w677]
                                tunnel: w433 -> [w676]
                                tunnel: w432 -> [w675]
                                tunnel: w431 -> [w674]
                                tunnel: [w668] -> w427
                                frame #0 {
                                # "valores voltaje"
                                # "mover polarizador"
                                # "crear grupo para guardar datos"
                                # "mover el polarizador"
                                n108 = invoke class="IntegratedStepperMotor" method="SetMoveAbsolutePosition"(reference=w480, error in=w479, "position"=w466) -> (reference out=w478:refnum<k24>, error out=w477:errorcluster)  [unwired: 1 in, 2 out]
                                n109 = invoke class="IntegratedStepperMotor" method="MoveAbsolute"(reference=w478, error in=w477, "waitTimeout"=0) -> (reference out=w475:refnum<k24>, error out=w474:errorcluster)  [unwired: 1 in, 2 out]
                                n110 = Number To Fractional String(number=w466) -> (F-format string=w469:string)  [unwired: 3 in]
                                n111 = Concatenate Strings("posición " ("string"), w469, "°" ("string")) -> (w467:string)
                                n112 = call <vilib>:"H5Gcreate.vi"("error in (no error)"=w464, "Name"=w467, "HDF5 Ref"=w465) -> ("error out"=w462:errorcluster, "HDF5 Group Ref"=w463:T13, "HDF5 Ref out"=w460:T13)  [unwired: 4 in]
                                n113 = invoke class="IntegratedStepperMotor" method="GetPositionCounter"(reference=w475, error in=w474) -> (reference out=w473:refnum<k24>, error out=w472:errorcluster, "GetPositionCounter"=→"Ángulo del polarizador":i32)  [unwired: 1 in]
                                }
                                frame #1 {
                                w493 = dbl[] []
                                # "mediciones de voltaje"
                                n114 = for {
                                tunnel: w494 -> [w518] mode=indexing
                                shift-right: [w498] -> w484
                                shift-left: w493 -> [w517]
                                shift-right: [w503] -> w483
                                shift-left: w493 -> [w505]
                                shift-right: [w497] -> w482
                                shift-left: w493 -> [w504]
                                shift-right: [w500] -> w481
                                shift-left: w493 -> [w515]
                                tunnel: w492 -> [w512]
                                tunnel: w491 -> [w510]
                                tunnel: [w496] -> w489
                                tunnel: [w495] -> w488
                                stop <- w519 stop-if-true
                                # "graficas"
                                n115 = flat-sequence {
                                tunnel: w518 -> [w529]
                                tunnel: [w524] -> w516
                                tunnel: [w523] -> w514
                                tunnel: [w522] -> w513
                                tunnel: w512 -> [w522]
                                tunnel: [w521] -> w511
                                tunnel: w510 -> [w521]
                                tunnel: [w520] -> w495
                                tunnel: w513 -> [w573]
                                tunnel: w511 -> [w572]
                                tunnel: [w568] -> w508
                                tunnel: [w567] -> w509
                                tunnel: [w566] -> w496
                                frame #0 {
                                n116 = local read "Config. voltaje y corriente"() -> (w528:T3)
                                n117 = flat-sequence {
                                tunnel: w529 -> [w544]
                                tunnel: w527 -> [w535]
                                tunnel: w525 -> [w543]
                                tunnel: [w533] -> w532
                                tunnel: [w538] -> w531
                                tunnel: [w537] -> w530
                                tunnel: w526 -> [w534]
                                tunnel: [w533] -> w524
                                tunnel: [w565] -> _
                                tunnel: w532 -> [w565]
                                tunnel: [w555] -> w523
                                tunnel: w531 -> [w557]
                                tunnel: w530 -> [w564]
                                tunnel: [w556] -> w520
                                frame #0 {
                                # "obtener valor  del voltaje"
                                n118 = call <instrlib>:"Initialize.vi"("VISA resource name"=refnum<visa-resource-name> refnum) -> ("error out"=w550:errorcluster, "VISA resource name out"=w551:refnum<visa-resource-name>)  [unwired: 9 in]
                                n119 = call <instrlib>:"Configure Output.vi"("VISA resource name"=w551, "Manual Range(0.00)"=w544, "Function(0:Voltage)"=w535, "Enable Output (T: Enable)"=TRUE, "error in (no error)"=w550, "Unit(V)"=w534) -> ("VISA resource name out"=w548:refnum<visa-resource-name>, "error out"=w547:errorcluster)  [unwired: 8 in]
                                n120 = flat-sequence {
                                tunnel: w547 -> [w553]
                                tunnel: [w553] -> w546
                                tunnel: w548 -> [w552]
                                tunnel: [w552] -> w538
                                frame #0 {
                                n121 = Wait (ms)(milliseconds to wait=u32 1000) -> ()  [unwired: 1 out]
                                }
                                }
                                n122 = call <instrlib>:"Read Output.vi"("VISA resource name"=w538, "Measurement Function (0:Voltage)"=w543, "error in (no error)"=w546) -> ("VISA resource name out"=w542:refnum<visa-resource-name>, "Measurement"=w545:string, "error out"=w541:errorcluster)  [unwired: 10 in]
                                n123 = Fract/Exp String To Number(string=w545) -> (number=w533:dbl)  [unwired: 3 in, 1 out]
                                n124 = call <instrlib>:"Error Query.vi"("error in (no error)"=w541, "VISA resource name"=w542) -> ("error out"=w540:errorcluster, "VISA resource name out"=w539:refnum<visa-resource-name>)  [unwired: 6 in, 2 out]
                                n125 = local write "Valor voltaje"(w533) -> ()
                                n126 = call <instrlib>:"Close.vi"("error in (no error)"=w540, "VISA resource name"=w539) -> ("error out"=w537:errorcluster)  [unwired: 9 in]
                                }
                                frame #1 {
                                w563 = u16 1 items=["Voltage", "Current", "Power"] ("Measurement Function (0:Voltage)")
                                # "corriente"
                                n127 = call <instrlib>:"Read Output.vi"("VISA resource name"=w557, "Measurement Function (0:Voltage)"=w563, "error in (no error)"=w564) -> ("VISA resource name out"=w559:refnum<visa-resource-name>, "Measurement"=w562:string, "error out"=w558:errorcluster)  [unwired: 10 in]
                                n128 = Fract/Exp String To Number(string=w562) -> (number=w555:dbl)  [unwired: 3 in, 1 out]
                                n129 = call <instrlib>:"Error Query.vi"("error in (no error)"=w558, "VISA resource name"=w559) -> ("error out"=w560:errorcluster, "VISA resource name out"=w561:refnum<visa-resource-name>)  [unwired: 6 in, 2 out]
                                n130 = local write "corriente"(w555) -> ()
                                n131 = call <instrlib>:"Close.vi"("error in (no error)"=w560, "VISA resource name"=w561) -> ("error out"=w556:errorcluster)  [unwired: 9 in]
                                }
                                }
                                n132 = Unbundle By Name(w528) -> ("Function(0:Voltage)"=w527:u16, "Unit(V)"=w526:u16, "Measurement Function (0:Voltage)"=w525:u16)
                                }
                                frame #1 {
                                # "adquisición de los datos"
                                n133 = local read "Powermeter"() -> (w577:T1)
                                n134 = local read "Config. fotodiodo"() -> (w582:cluster{"tiempo. lect.":dbl, "num. med":dbl})
                                n135 = Unbundle By Name(w577) -> ("Readout Config"=w574:string, "tiempo. lect."=w576:dbl, "average rate"=w575:dbl)
                                n136 = Unbundle By Name(w582) -> ("tiempo. lect."=w581:dbl, "num. med"=w580:dbl)
                                n137 = To Long Integer(number=w576) -> (32bit integer=w571:i32)
                                n138 = To Long Integer(number=w575) -> (32bit integer=w570:i32)
                                n139 = To Long Integer(number=w580) -> (32bit integer=w579:i32)
                                n140 = To Long Integer(number=w581) -> (32bit integer=w578:i32)
                                n141 = for {
                                N: w579 -> [w598]
                                shift-right: [w586] -> _
                                shift-left: enum16{"0", "1", "2"}."0" ("f") -> [w600]
                                tunnel: w573 -> [w602]
                                tunnel: w572 -> [w601]
                                shift-right: [w595] -> w568
                                shift-left: _ -> [w594]
                                tunnel: [w583] -> w567 mode=indexing
                                tunnel: w574 -> [w592]
                                tunnel: w571 -> [w591]
                                tunnel: w570 -> [w590]
                                tunnel: w578 -> [w589]
                                tunnel: [w588] -> _
                                tunnel: [w587] -> w566
                                i -> [w597]
                                w593 = u16 0 items=["LockIn", "LockIn-DMM"] ("Tipo")
                                n142 = Increment(x=w597) -> (x+1=w596:i32)
                                n143 = Wait (ms)(milliseconds to wait=w589) -> ()  [unwired: 1 out]
                                n144 = Greater Or Equal?(x=w598, y=w596) -> (x >= y?=w599:bool)
                                n145 = call "25_P-GPIB-LockIn510.vi"("Tipo"=w593, "P-DMM"="1:16", "P-LockIn"="1:3") -> ("LockIn"=w583:dbl)  [unwired: 1 in, 1 out]
                                n146 = local write "LockIn"(w583) -> ()
                                n147 = case shown="\"2\"" w600 {
                                tunnel: w602 -> [w613 w629 w656]
                                tunnel: w601 -> [w608 w628 w655]
                                tunnel: [enum16{"0", "1", "2"}."1" w623 enum16{"0", "1", "2"}."0"] -> w586
                                tunnel: [w606 w625 w654] -> w588
                                tunnel: [w605 w624 w649] -> w587
                                tunnel: w599 -> [_ w619 _]
                                tunnel: w594 -> [w604 w618 w648]
                                tunnel: [w604 w618 w646] -> w595
                                tunnel: w592 -> [_ w617 w645]
                                tunnel: w591 -> [_ w616 _]
                                tunnel: w590 -> [w603 _ _]
                                frame "0", Default {
                                # "Query errors"
                                # "Example: setting the averaging rate"
                                # "Measurement Configuration\nUse this frame to set the measurement relevant parameters\ne.g. wavelength, measurement range, bandwidth etc."
                                n148 = Number To Decimal String(number=w603) -> (decimal integer string=w614:string)  [unwired: 1 in]
                                n149 = Concatenate Strings("SENS:AVER " ("string"), w614) -> (w612:string)
                                n150 = call "PM100D_Write.vi"("error in (no error)"=w608, "Command"=w612, "VISA in"=w613) -> ("error out"=w609:errorcluster, "VISA out"=w611:refnum<visa-resource-name>)
                                n151 = call "PM100D_SYST-ERR.vi"("error out 2"=w609, "VISA In"=w611) -> ("error out"=w605:errorcluster, "Error"=→"Error log":string, "VISA Out"=w606:refnum<visa-resource-name>)  [unwired: 1 in]
                                }
                                frame "1" {
                                # "Measurement Value Selection"
                                n152 = call "PM100D_ConfMeas.vi"("error in"=w628, "Conf:"=w617, "VISA In"=w629) -> ("error out"=w626:errorcluster, "dup VISA session"=w627:refnum<visa-resource-name>)
                                n153 = while {
                                tunnel: w627 -> [w639]
                                tunnel: w626 -> [w638]
                                tunnel: [w637] -> w625
                                tunnel: [w636] -> w624
                                tunnel: [w632] -> w620
                                tunnel: w619 -> [w631]
                                tunnel: w616 -> [w630]
                                i -> [w634]
                                stop <- w635 stop-if-true
                                # "Query Operation Register for new data"
                                n154 = call "PM100D_Read.vi"("error in (no error)"=w638, "Command"="STAT:OPER?", "VISA in"=w639) -> ("error out"=w636:errorcluster, "ReadValue"=w642:string, "VISA out"=w637:refnum<visa-resource-name>)  [unwired: 1 in]
                                n155 = Decimal String To Number(string=w642) -> (number=w641:i32)  [unwired: 2 in, 1 out]
                                n156 = Equal?(x=w641, y=512) -> (x = y?=w632:bool)
                                "New" <- w632
                                n157 = Equal?(x=w630, y=w634) -> (x = y?=w633:bool)
                                n158 = Compound Arithmetic op=OR(w632, w633, w631) -> (w635:bool)
                                }
                                n159 = Select(t=enum16{"0", "1", "2"}."2", s=w620, f=enum16{"0", "1", "2"}."1") -> (s? t:f=w623:enum16{"0", "1", "2"})
                                }
                                frame "2" {
                                n160 = case shown="\"POW\", Default" w645 {
                                tunnel: ["W" "A" "V" "J" "Hz" "W/cm²" "J/cm²" "Ohm" "°C"] -> w651
                                frame "POW", Default {
                                }
                                frame "CURR" {
                                }
                                frame "VOLT" {
                                }
                                frame "ENER" {
                                }
                                frame "FREQ" {
                                }
                                frame "PDEN" {
                                }
                                frame "EDEN" {
                                }
                                frame "RES" {
                                }
                                frame "TEMP" {
                                }
                                }
                                n161 = call "PM100D_Read.vi"("error in (no error)"=w655, "Command"="FETC?", "VISA in"=w656) -> ("error out"=w649:errorcluster, "ReadValue"=w653:string, "VISA out"=w654:refnum<visa-resource-name>)  [unwired: 1 in]
                                n162 = Fract/Exp String To Number(use system decimal point (T)=FALSE, string=w653) -> (number=w647:dbl)  [unwired: 2 in, 1 out]
                                "valor potenciometro" <- w647
                                n163 = Format Into String(format string="%.;%_4p%s", w647, w651) -> (resulting string=→"Readout string":string)  [unwired: 2 in, 1 out]
                                n164 = Build Array (concatenate)(w648, w647) -> (w646:dbl[])
                                }
                                }
                                }
                                }
                                }
                                n165 = Build Array (concatenate)(w517, w516) -> (w498:dbl[])
                                n166 = Build Array (concatenate)(w515, w514) -> (w500:dbl[])
                                n167 = local read "stop medición"() -> (w519:bool)
                                n168 = call-poly <vilib>:"Mean.vi"("X"=w509) -> ("mean"=w507:dbl)  [unwired: 1 out]
                                n169 = call-poly <vilib>:"Mean.vi"("X"=w508) -> ("mean"=w506:dbl)  [unwired: 1 out]
                                n170 = Build Array (concatenate)(w504, w506) -> (w497:dbl[])
                                n171 = Build Array (concatenate)(w505, w507) -> (w503:dbl[])
                                n172 = Bundle(w498, w497) -> (→"Power meter":cluster{dbl[], dbl[]})  [unwired: 1 in]
                                n173 = Bundle(w498, w503) -> (→"Fototubo":cluster{dbl[], dbl[]})  [unwired: 1 in]
                                n174 = Bundle(w498, w500) -> (→"I-V":cluster{dbl[], dbl[]})  [unwired: 1 in]
                                }
                                }
                                frame #2 {
                                # "error mov polarizador"
                                # "error voltaje"
                                # "error potenciometro"
                                # "guardado de datos"
                                n175 = Build Array(w677, w676, w675, w674) -> (w671:dbl[][])
                                n176 = xnode "Simple H5Dwrite"("error in (no error)"=w669, "HDF5 Path or Ref"=w670, "Data"=w671) -> ("HDF5 Ref out"=w673:T13, "error out"=w672:errorcluster)  [unwired: 5 in, 1 out]
                                n177 = call <vilib>:"H5Gclose.vi"("error in (no error)"=w672, "HDF5 Group Ref"=w673) -> ("error out"=w668:errorcluster)  [unwired: 7 in]
                                }
                                }
                              }
                            }
                            frame #4 {
                              # "cerracdo de grupo y mov de polarizador"
                              n178 = invoke class="CageRotatorControl" method="CloseDevice"(reference=w890, error in=w891) -> (error out=w889:errorcluster)  [unwired: 1 in, 2 out]
                              n179 = call <vilib>:"H5Gclose.vi"("error in (no error)"=w886, "HDF5 Group Ref"=w885) -> ("error out"=w884:errorcluster)  [unwired: 7 in]
                            }
                          }
                        }
                      }
                    }
                    frame #2 {
                      # "detener medición"
                      n180 = local read "tipo"() -> (w899:enum16{"barrido", "manual"})
                      n181 = Equal?(x=w899, y=enum16{"barrido", "manual"}."manual") -> (x = y?=w900:bool)
                      n182 = case shown="False" w900 {
                        tunnel: [w904 TRUE] -> w897
                        tunnel: w896 -> [w907 _]
                        frame False {
                          n183 = Equal?(x=w907, y=6) -> (x = y?=w905:bool)
                          n184 = case shown="False" w905 {
                            tunnel: [FALSE TRUE] -> w904
                            frame False {
                            }
                            frame True {
                              n185 = One Button Dialog(message="Fin de Medición") -> ()  [unwired: 1 in, 1 out]
                            }
                          }
                        }
                        frame True {
                          n186 = One Button Dialog(message="Fin de Medición") -> ()  [unwired: 1 in, 1 out]
                        }
                      }
                    }
                  }
                  n187 = local read "stop"() -> (w108:bool)
                  n188 = Or(x=w106, y=w108) -> (x .or. y?=w107:bool)
                }
              }
              frame #2 {
                # "cierra archivo"
                n189 = call <vilib>:"H5Fclose.vi"("error in (no error)"=w918, "HDF5 Ref"=w917) -> ("error out"=w916:errorcluster)  [unwired: 7 in]
              }
            }
          }
        }
        n190 = call <vilib>:"IMAQdx Grab2.vi"("error in"=w43, "Image In"=w42, "Session In"=w44) -> ("error out"=w41:errorcluster, "Image Out"=w39:T4, "Session Out"=w40:T5)  [unwired: 5 in, 1 out]
        "Imágen" <- w39
      }
    }
  }
  n191 = call <vilib>:"IMAQdx Close Camera.vi"("error in"=w8, "Session In"=w6) -> ("error out"=w9:errorcluster)  [unwired: 9 in]
  n192 = call "IMAQ Dispose"("Image"=w7, "error in (no error)"=w9) -> ("error out"=w1:errorcluster)  [unwired: 4 in]
  n193 = Merge Errors(w2, w3, w4, w1) -> (w5:errorcluster)
  n194 = call <vilib>:"General Error Handler.vi"("error in (no error)"=w5) -> ()  [unwired: 10 in, 5 out]
